vi "MultirunBuilderForNamedLocations3.vi"() -> ()   [LabVIEW 2015]
uses:
  MultirunBuilderSubVIs/RowTemplate.ctl
  Anemometry Sub Vis/Gen Trav/Spacing.ctl
  Anemometry Sub Vis/Controls/Multi_run_mode.ctl
  MultirunBuilderSubVIs/ReformattedTaskArray.ctl
  Anemometry Sub Vis/Controls/Tunnel_Coordinates.ctl
  MultirunBuilderSubVIs/Set Speed Only.vi
  MultirunBuilderSubVIs/Wait (minutes).vi
  MultirunBuilderSubVIs/Single Measurement.vi
  MultirunBuilderSubVIs/Auto Calibrate.vi
  MultirunBuilderSubVIs/MoveTT.vi
  Anemometry Sub Vis/Globals/Meas_global.vi
  Anemometry Sub Vis/File/Setup_Filetype.ctl
panel:
  in  "Generate Cmd File":bool
  in  "Tab Control":enum32{"Globals", "Task Array", "Dev"}(tab)
  in  "TaskArray":T1 {"Carrier_2 Q (l/min)" format="%#.2f"; "Row Duration (mins)" format="%#.1f min"; "Row No" min=0 format="row %.0f"; "Trace Gas Concentration (%)" min=0.0 format="%#_4f"; "Carrier_1 Q (l/min)" format="%#.2f"; "Tunnel Speed" format="%#.2f m/s"; "Start X" format="%#.2f"; "Start Y" format="%#.2f"; "Start Z" format="%#.2f"; "End X" format="%#.2f"; "End Y" format="%#.2f"; "End Z" format="%#.2f"; "No. of pts." format="%.0f pts"; "Averaging time (min)" min=0.0 format="%#.2f min"}
  out "Startup Index":bool
  in  "Re-initialize":bool
  in  "Stop Button":bool
  in  "RowTemplate":T3 {"Carrier_2 Q (l/min)" format="%#.2f"; "Row Duration (mins)" format="%#.1f"; "Row No" min=0; "Trace Gas Concentration (%)" min=0.0 format="%#_4f"; "Carrier_1 Q (l/min)" format="%#.2f"; "Tunnel Speed" format="%#.2f"; "Start X" format="%#.2f"; "Start Y" format="%#.2f"; "Start Z" format="%#.2f"; "End X" format="%#.2f"; "End Y" format="%#.2f"; "End Z" format="%#.2f"; "Averaging time (min)" min=0.0 format="%#.2f"}
  # "X           Y            Z"
  # "Start"
  # "End"
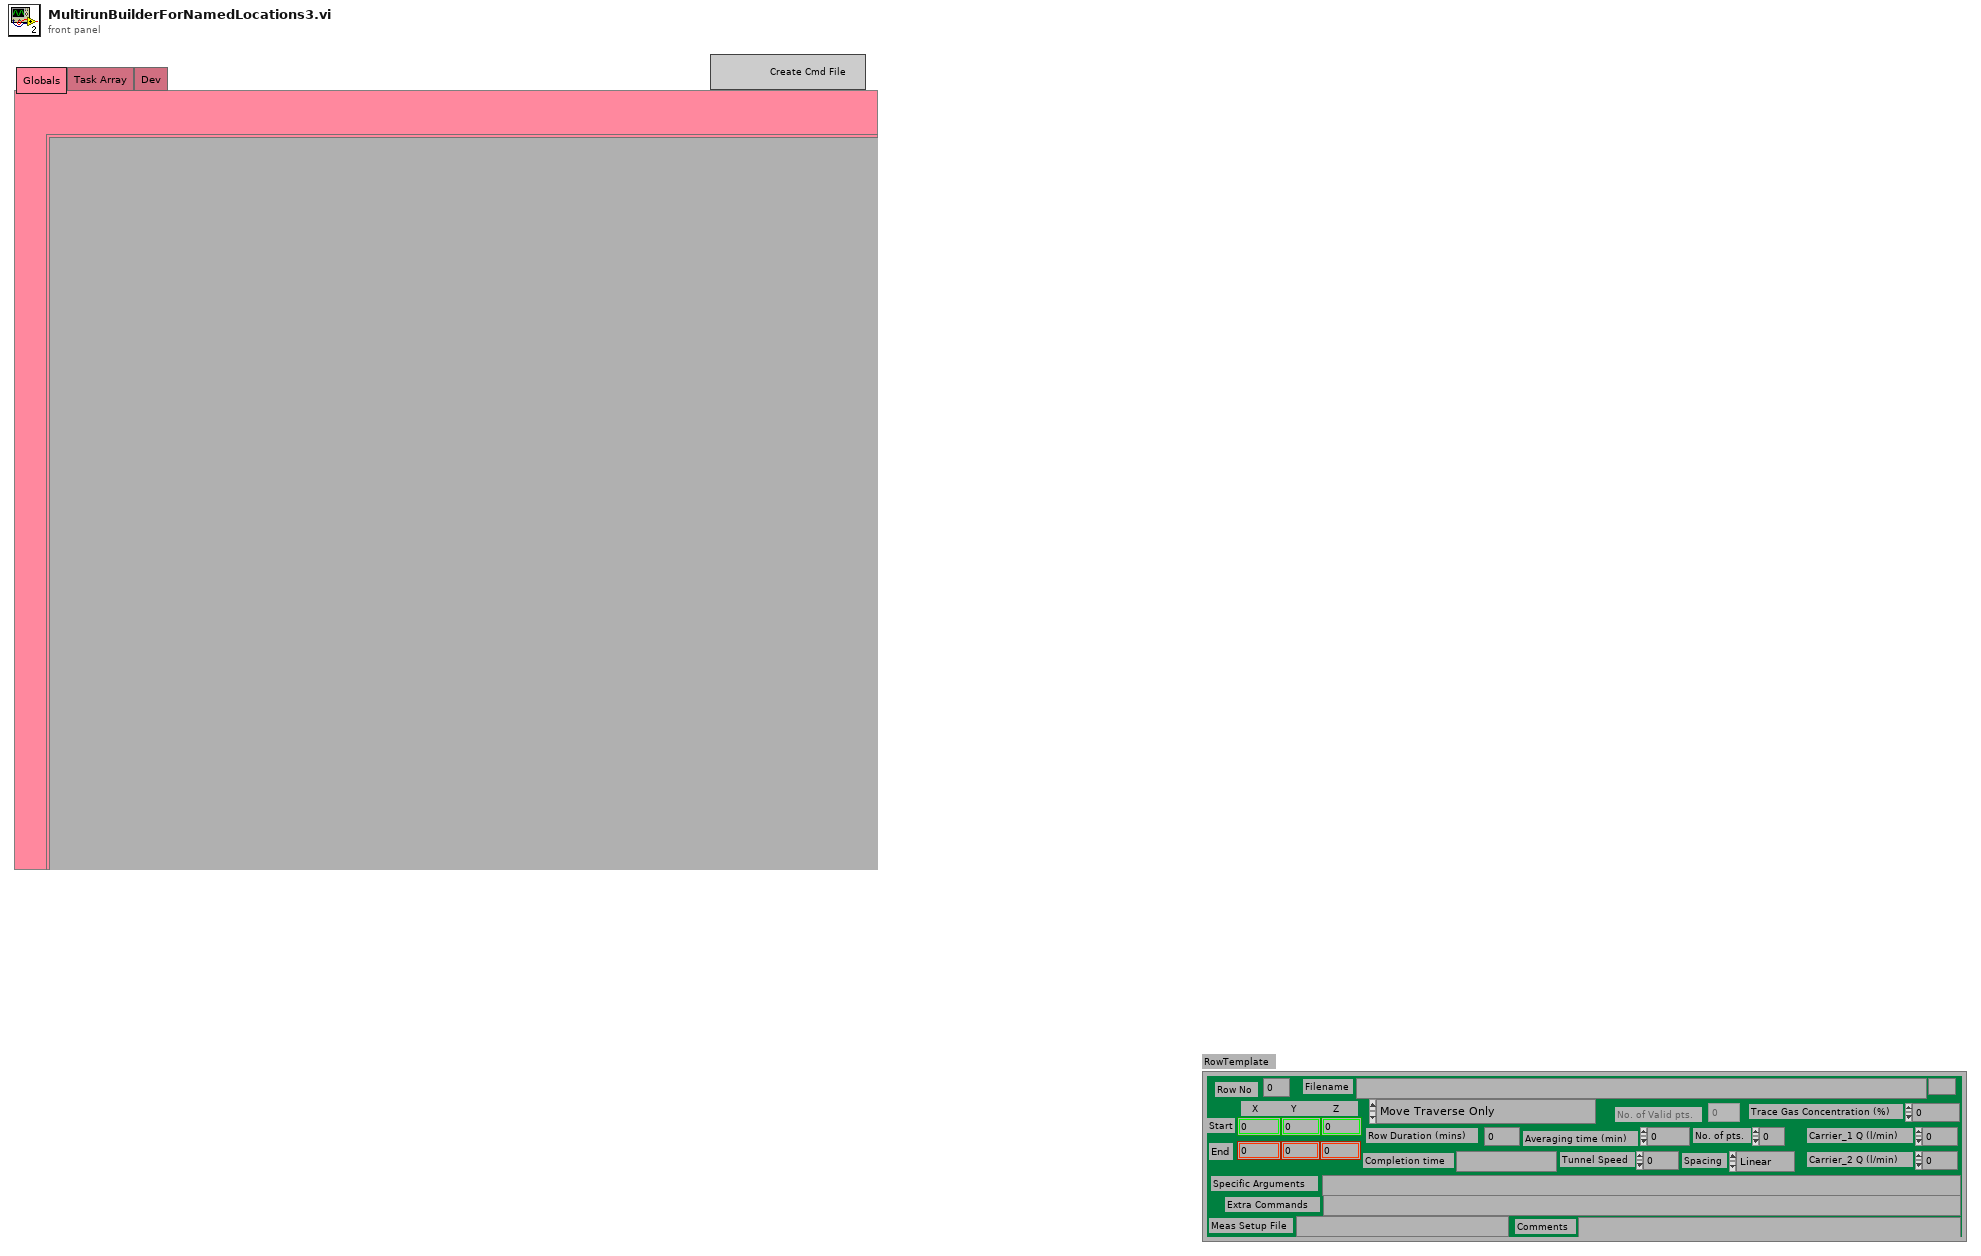
[diagram p1: front panel]
types:
  T1 = typedef "ReformattedTaskArray.ctl" = cluster{"Start X":sgl, "Start Y":sgl, "Start Z":sgl, "End X":sgl, "End Y":sgl, "End Z":sgl, "No. of pts.":i32, "Spacing":T2, "Filename":path, "Tunnel Speed":dbl, "Averaging time (min)":dbl, "Extra Commands":string, "Carrier_1 Q (l/min)":dbl, "Carrier_2 Q (l/min)":dbl, "Trace Gas Concentration (%)":dbl, "Specific Arguments":string, "Comments":string, "Row No":i32, "Row Type Selector":enum16{"Move Traverse Only", "Set Tunnel Speed Only", "Set Source Only", "Set Measurement Conditions", "Single Measurement", "Vertical Profile", "Lateral Profile", "Longitudinal Profile", "Explore Volume", "Multi-Axis Profile", "Auto Calibrate", "Meas Fast FID Bkgnd", "Check Beam Power", "Scanning Valve Measurement", "Run VI Named:", "Set ADAM Ch", "Wait (minutes)", "Send Message", "Synchronize With:", "Fall Back to this Row", "Turn Off Row Repeating", "Blank Row", "Traverse 3D Volume"}, "Completion time":string, "Row Duration (mins)":dbl, "No. of Valid pts.":i32, "Meas Setup File":string}[]
  T2 = typedef "Spacing.ctl" = enum16{"Linear", "Log", "Gauss", "Specified", "N/A"}
  T3 = typedef "RowTemplate.ctl" = cluster{"Start X":sgl, "Start Y":sgl, "Start Z":sgl, "End X":sgl, "End Y":sgl, "End Z":sgl, "No. of pts.":i32, "Spacing":T2, "Filename":path, "Tunnel Speed":dbl, "Averaging time (min)":dbl, "Extra Commands":string, "Carrier_1 Q (l/min)":dbl, "Carrier_2 Q (l/min)":dbl, "Trace Gas Concentration (%)":dbl, "Specific Arguments":string, "Comments":string, "Row No":i32, "Row Type Selector":T4, "Completion time":string, "Row Duration (mins)":dbl, "No. of Valid pts.":i32, "Meas Setup File":string}
  T4 = typedef "Multi_run_mode.ctl" = enum16{"Move Traverse Only", "Set Tunnel Speed Only", "Set Source Only", "Set Measurement Conditions", "Single Measurement", "Vertical Profile", "Lateral Profile", "Longitudinal Profile", "Explore Volume", "Multi-Axis Profile", "Auto Calibrate", "Meas Fast FID Bkgnd", "Check Beam Power", "Scanning Valve Measurement", "Run VI Named:", "Set ADAM Ch", "Wait (minutes)", "Send Message", "Synchronize With:", "Fall Back to this Row", "Turn Off Row Repeating", "Blank Row", "Traverse 3D Volume"}
  T5 = cluster{"Azimuth Array Index":u32, "Vert Prof Array Index":u32, "Lat Prof Array Index":u32, "Azimuth Array Index 2":u32}
  T6 = cluster{"X":dbl, "Y":dbl, "Z":dbl, string, "Use Tunnel Coords?":bool}
  T7 = enum16{"Load Command File", "Save Command File", "Check Multi Run Prog", "Check Multi Run Prog With Live Moves", "Run Multi Run Prog"}
  T8 = typedef "Tunnel_Coordinates.ctl" = enum16{"Work in Tunnel Coordinates", "Work in Model Coordinates"}
  T9 = cluster{"Tunnel Warm Up":bool, "AutoCal":bool, "Zeroes 2":bool, "Turn Table Schedule":bool, "Global Cal Checks":bool, "Local Cal Checks":bool, "Vertical Profile":bool, "Lateral Profile":bool, "Reinitialize Task Array":bool, "Save Command File":bool, "Longitudinal Profile":bool}
  T10 = typedef "CorrectionsCluster.ctl" = cluster{"Use Height Corrections":bool, "TT.Azimuths":dbl[], "Z.HeightCorrs":dbl[][], "Corrections from File":bool, "Height Survey Filepaths":path[]}
  T11 = cluster{"Start X":sgl, "Start Y":sgl, "Start Z":sgl, "End X":sgl, "End Y":sgl, "End Z":sgl, "No. of pts.":i32, "Spacing":T2, "Filename":path, "Tunnel Speed":dbl, "Averaging time (min)":dbl, "Extra Commands":string, "Carrier_1 Q (l/min)":dbl, "Carrier_2 Q (l/min)":dbl, "Trace Gas Concentration (%)":dbl, "Specific Arguments":string, "Comments":string, "Row No":i32, "Row Type Selector":T4, "Completion time":string, "Row Duration (mins)":dbl, "No. of Valid pts.":i32, "Meas Setup File":string}[]
  T12 = typedef "SingleMeas_Repeater.ctl" = cluster{"X":dbl, "Y":dbl, "Z":dbl, "Use Tunnel Coords?":bool, "RepeatEveryXDeg":dbl}
  T13 = typedef "MRBRowTaskSelector.ctl" = enum16{"Move Traverse Only", "Set Tunnel Speed Only", "Set Source Only", "Set Measurement Conditions", "Single Measurement", "Vertical Profile", "Lateral Profile", "Longitudinal Profile", "Explore Volume", "Multi-Axis Profile", "Auto Calibrate", "Meas Fast FID Bkgnd", "Check Beam Power", "Scanning Valve Measurement", "Run VI Named:", "MoveTT", "TravZSurvey", "Set ADAM Ch", "Wait (minutes)", "Send Message", "Synchronize With:", "Fall Back to this Row", "Turn Off Row Repeating", "Blank Row", "Traverse 3D Volume"}
  T14 = cluster{"Row Type Selector":T13, "Index":dbl, "Direction":enum16{"Forward", "Reverse"}}[]
  T15 = cluster{"Tunnel Off":bool, "Local Cal Checks":bool, "Global Cal Checks":bool, "Zeroes":bool, "AutoCal":bool, "Turn Table --> Zero":bool}
  T16 = typedef "Setup_Filetype.ctl" = enum16{"Measurement Setups", "Calibration Setups", "General", "Results File Plotter Setups", "Speed Calib Tweaks"}
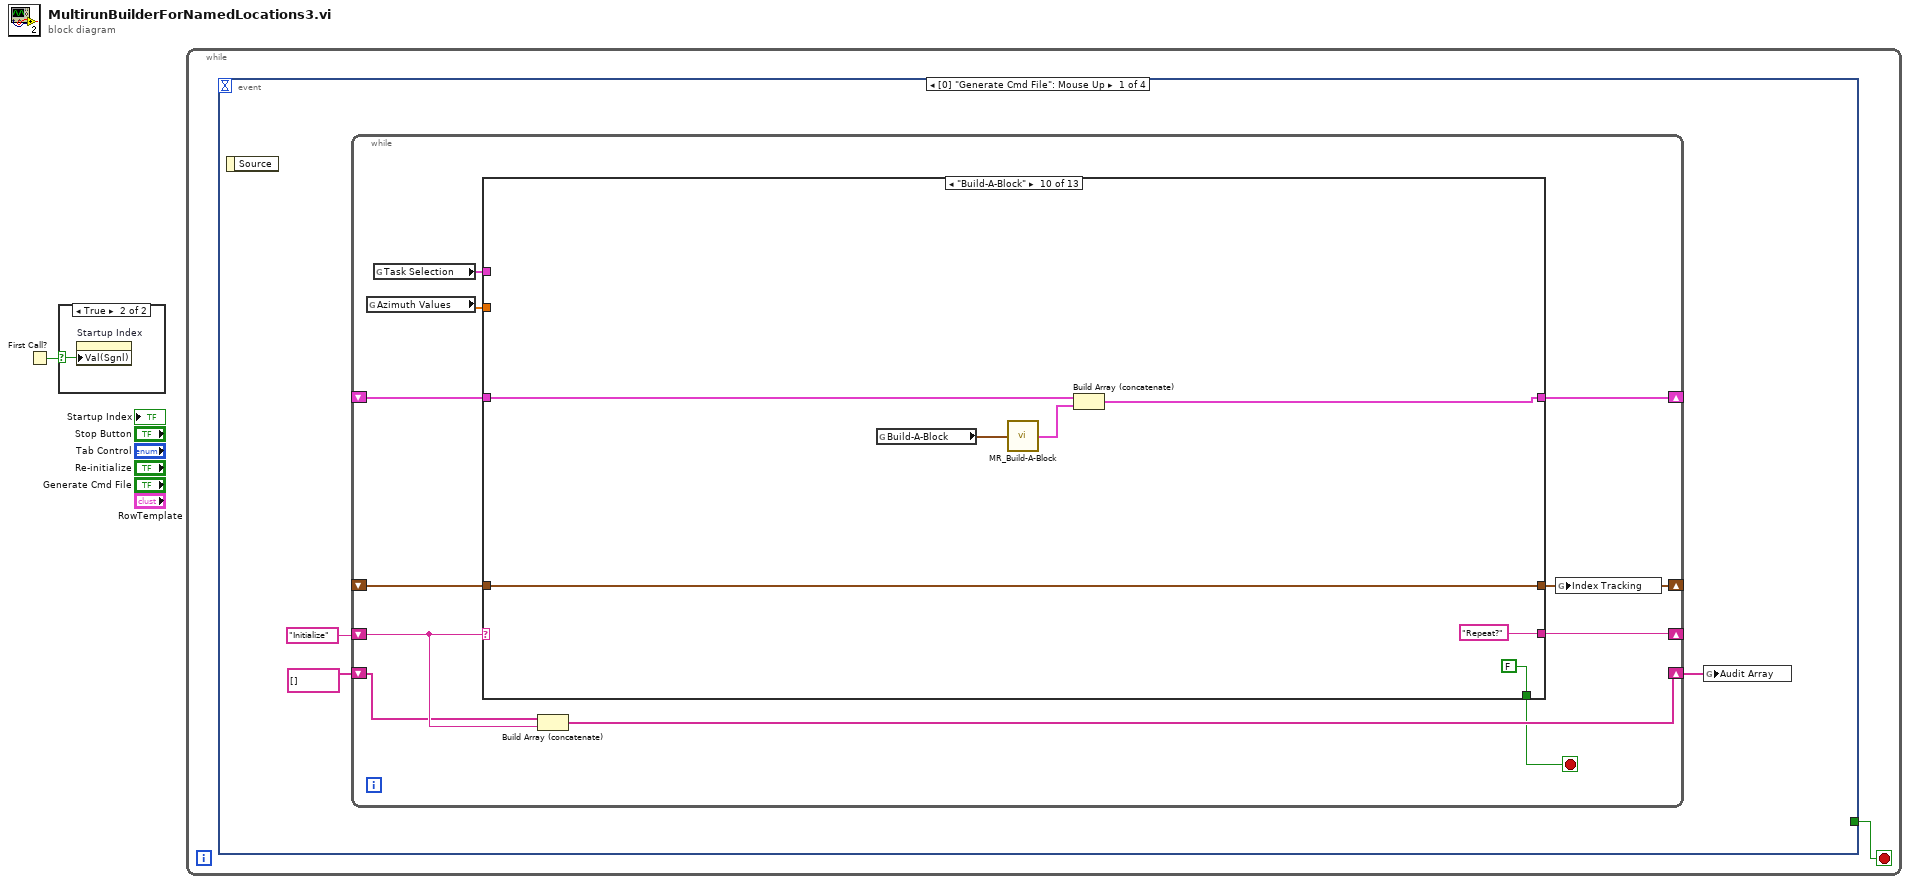
[diagram p0: block diagram]
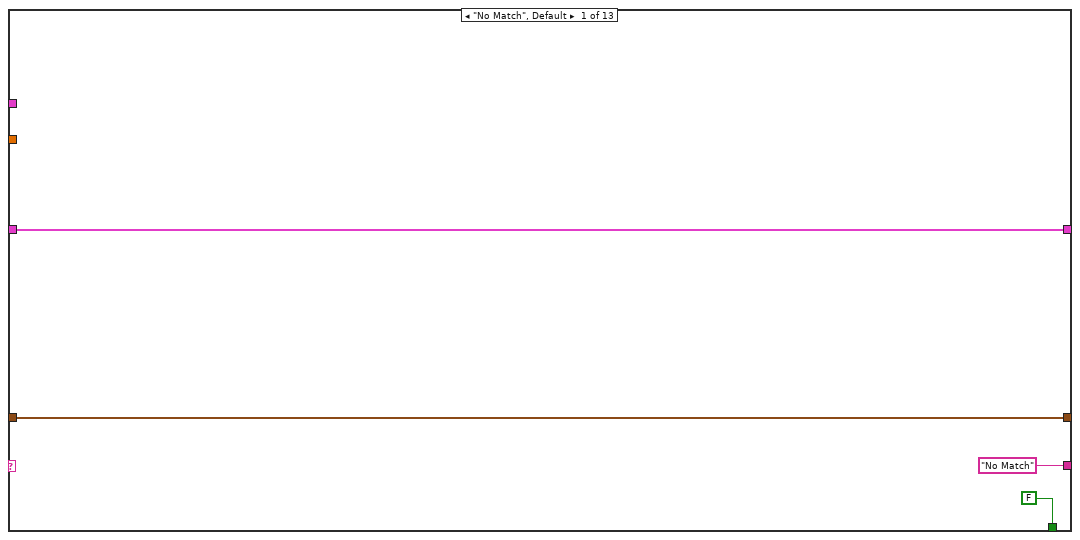
[diagram p2: hidden frame]
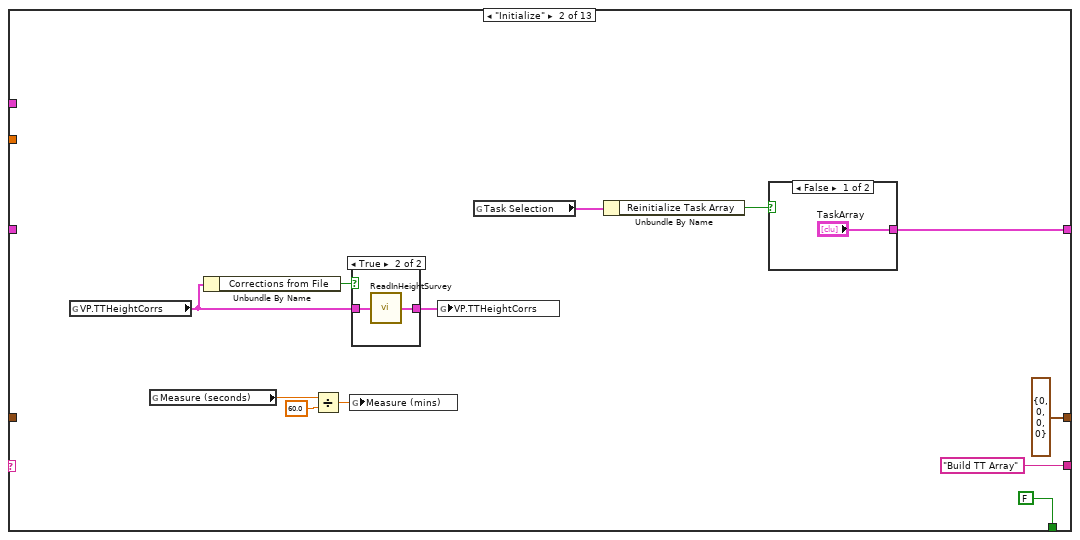
[diagram p3: hidden frame]
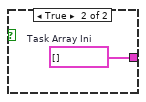
[diagram p5: hidden frame]
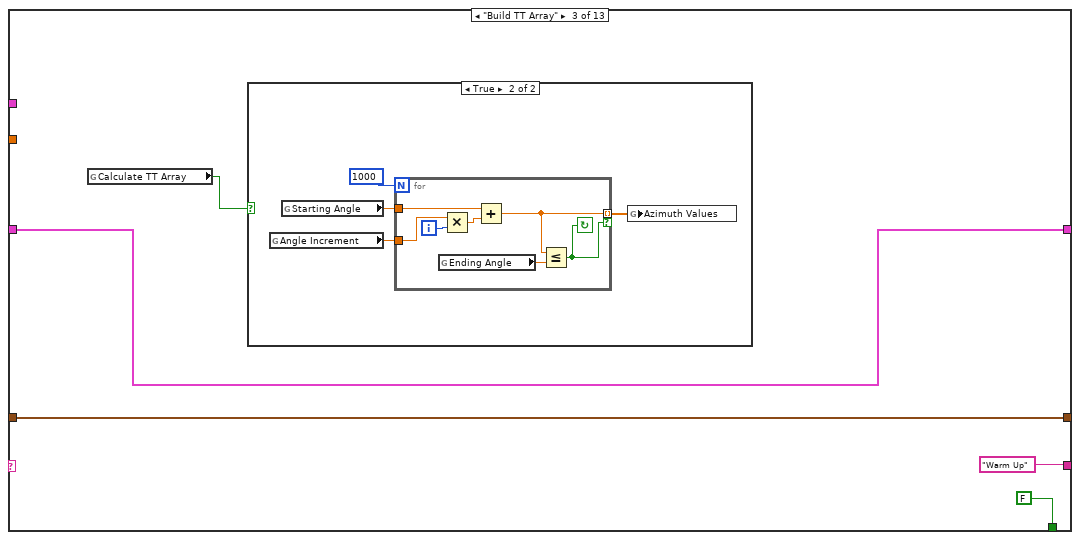
[diagram p6: hidden frame]
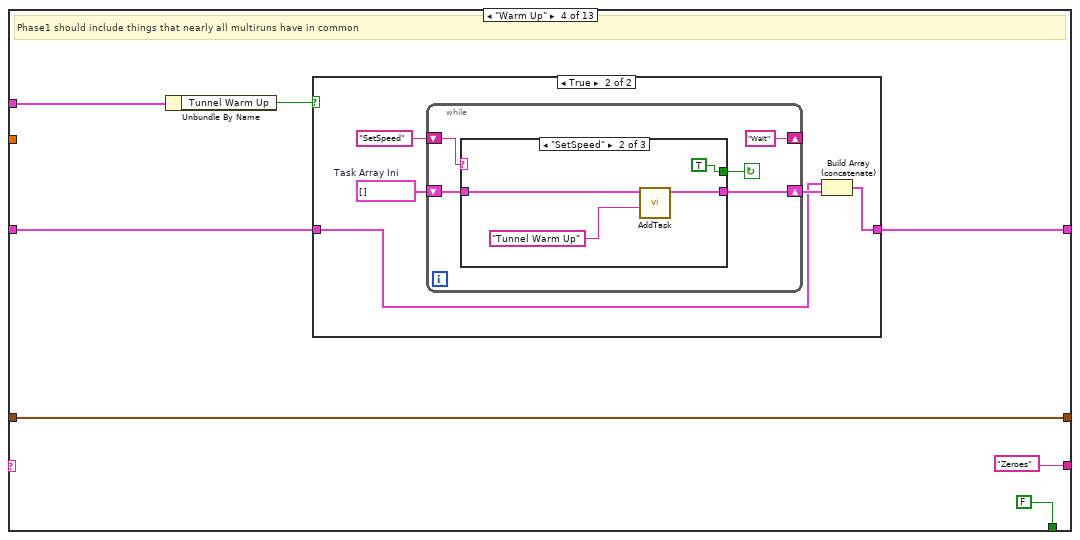
[diagram p8: hidden frame]
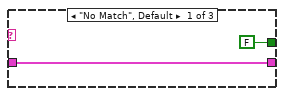
[diagram p10: hidden frame]
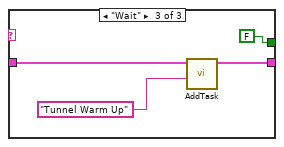
[diagram p11: hidden frame]
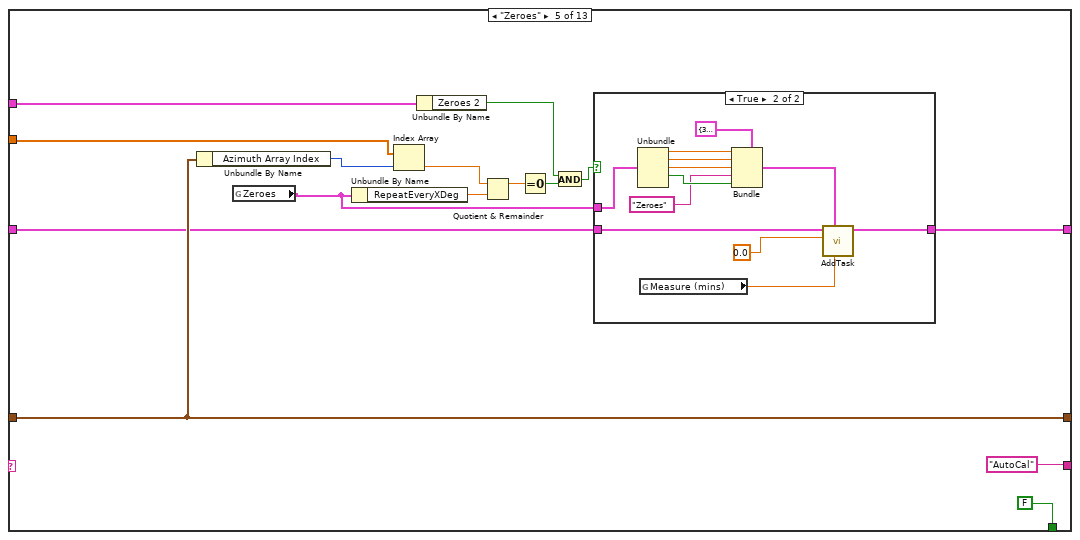
[diagram p12: hidden frame]
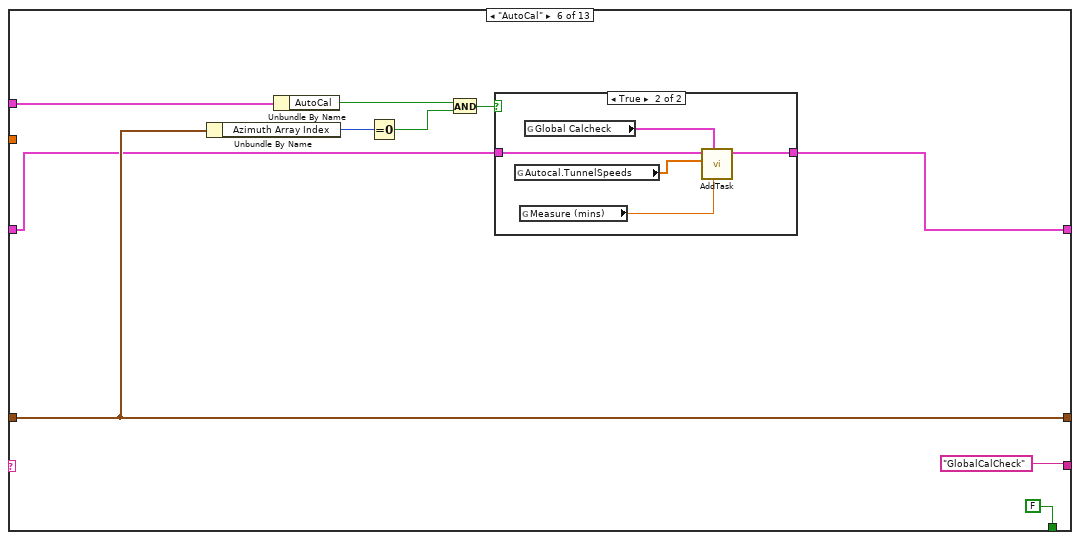
[diagram p14: hidden frame]
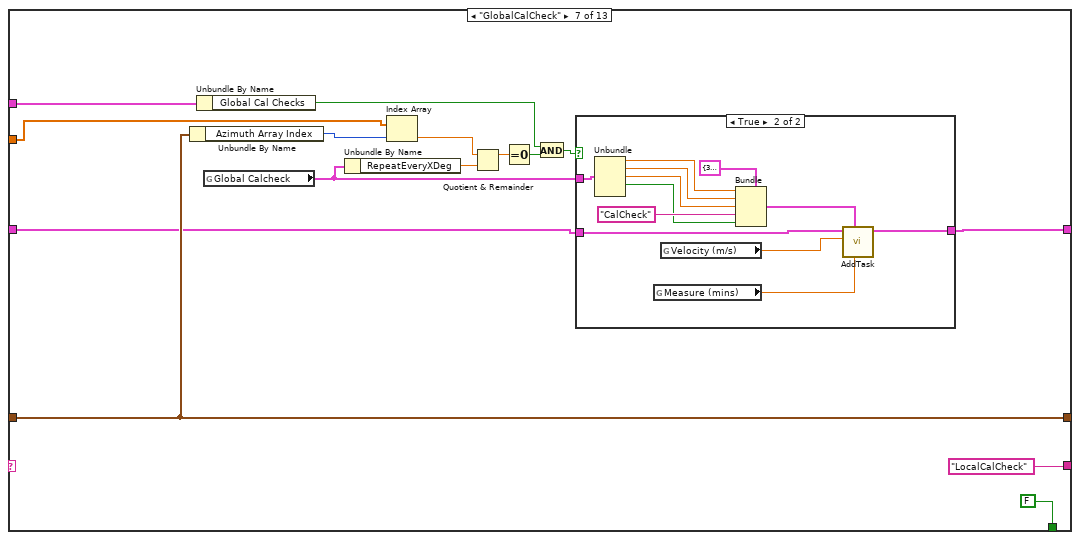
[diagram p16: hidden frame]
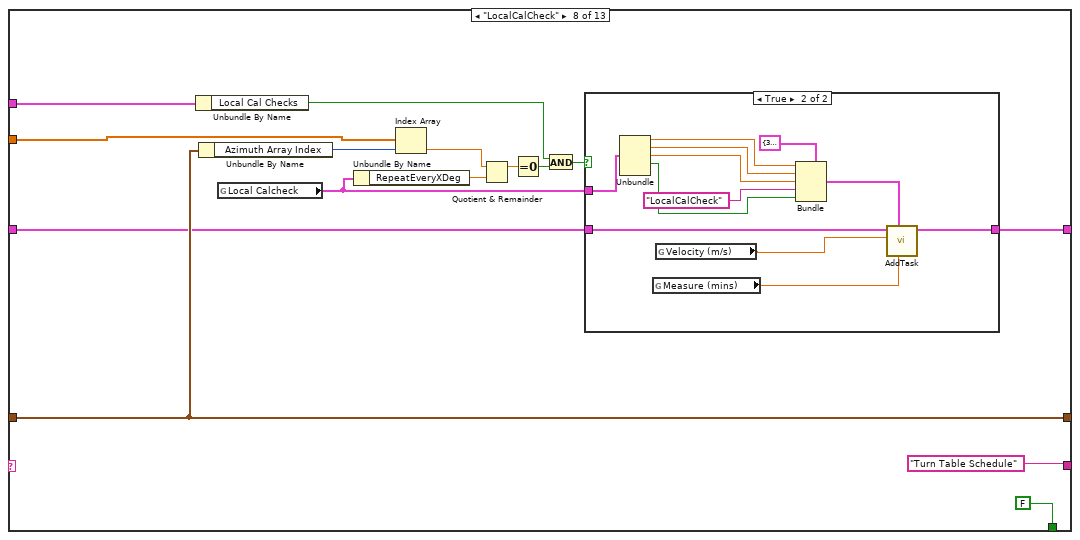
[diagram p18: hidden frame]
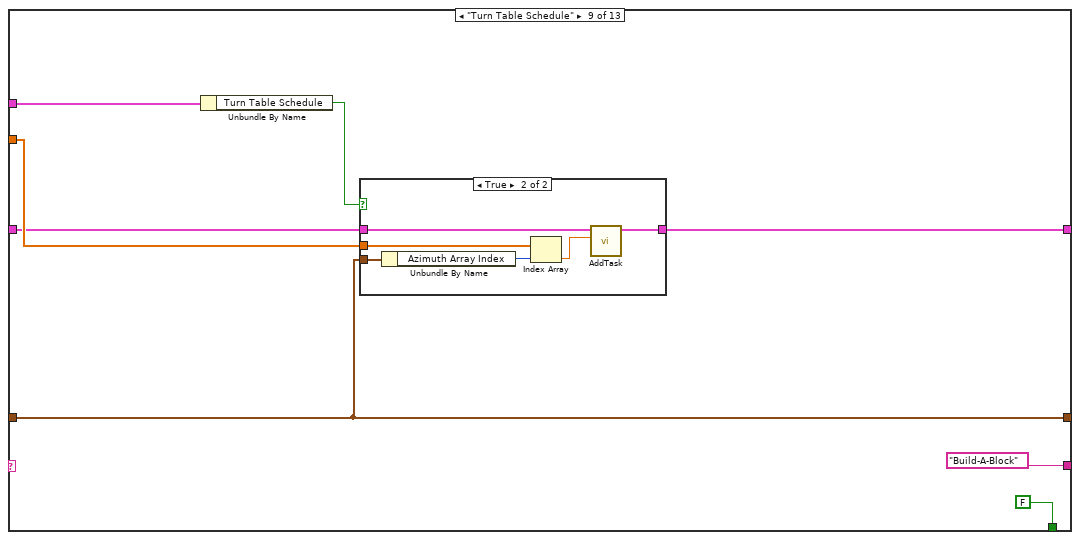
[diagram p20: hidden frame]
diagram:
  n1 = First Call?() -> (First Call?: T/F=w1:bool)
  n2 = case shown="True" w1 {
    selector: w1 -> [_ w2]
    frame False {
    }
    frame True {
      n3 = property on="Startup Index" class="Bool (strict)"("Val(Sgnl)"=w2) -> ()  [unwired: 2 in, 2 out]
    }
  }
  n4 = while {
    stop <- w3 stop-if-true
    n5 = event shown="[0] \"Generate Cmd File\": Mouse Up" {
      selector: _ -> [_ _ _ _]
      dyn-events: _ -> [_ _ _ _]
      timeout: _ -> [_ _ _ _]
      tunnel: [_ _ _ TRUE] -> w3
      event "Generate Cmd File": Mouse Up {
        n6 = event-data() -> ()  [unwired: 1 in, 1 out]
        n7 = while {
          shift-right: [w17] -> _
          shift-left: "Initialize" -> [w15]
          shift-right: [w10] -> _
          shift-left: _ -> [w11]
          shift-right: [w14] -> w6
          shift-left: string[] [] -> [w13]
          shift-right: [w9] -> _
          shift-left: _ -> [w16]
          stop <- w12 stop-if-true
          n8 = global read "MRCMDFBGlobal.vi" "Azimuth Values"() -> (w7:dbl[])
          n9 = global read "MRCMDFBGlobal.vi" "Task Selection"() -> (w8:T9)
          n10 = case shown="\"Build-A-Block\"" w15 {
            tunnel: ["No Match" "Build TT Array" "Warm Up" "Zeroes" "AutoCal" "GlobalCalCheck" "LocalCalCheck" "Turn Table Schedule" "Build-A-Block" "Repeat?" w209 "Save Multirun?" ("t") _] -> w17
            tunnel: [FALSE ("Stop Button") FALSE ("Stop Button") FALSE ("Stop Button") FALSE ("Stop Button") FALSE ("Stop Button") FALSE ("Stop Button") FALSE ("Stop Button") FALSE ("Stop Button") FALSE ("Stop Button") FALSE ("Stop Button") FALSE ("Stop Button") FALSE TRUE] -> w12
            tunnel: w7 -> [_ _ _ _ w95 _ w131 w158 w189 _ w208 _ _]
            tunnel: w16 -> [w19 _ w42 w59 w93 w117 w134 w163 w185 w199 w214 w242 w342]
            tunnel: [w19 T5 {"Azimuth Array Index"=0, "Vert Prof Array Index"=0, "Lat Prof Array Index"=0, "Azimuth Array Index 2"=0} ("Index Tracking") w42 w59 w93 w117 w134 w163 w185 w199 w212 w242 w342] -> w9
            tunnel: w8 -> [_ _ _ w58 w89 w113 w133 w162 w186 _ w205 _ w346]
            tunnel: w11 -> [w18 _ w40 w56 w84 w111 w128 w157 w184 w201 w206 w233 w344]
            tunnel: [w18 w28 w40 w55 w85 w112 w129 w156 w183 w200 w206 w234 w340] -> w10
            frame "No Match", Default {
            }
            frame "Initialize" {
              n11 = global read "MRCMDFBGlobal.vi" "VP.TTHeightCorrs"() -> (w25:T10)
              n12 = global read "MRCMDFBGlobal.vi" "Measure (seconds)"() -> (w22:dbl)
              n13 = Unbundle By Name(w25) -> ("Corrections from File"=w27:bool)
              n14 = Divide(x=w22, y=60.0 ("x")) -> (x/y=w23:dbl)
              n15 = global write "MRCMDFBGlobal.vi" "Measure (mins)"(w23) -> ()
              n16 = case shown="True" w27 {
                tunnel: w25 -> [w34 w36]
                tunnel: [w34 w35] -> w26
                frame False {
                }
                frame True {
                  n17 = call "ReadInHeightSurvey.vi"("VP.TTHeightCorrs In"=w36) -> ("VP.TTHeightCorrs Out"=w35:T10)
                }
              }
              n18 = global write "MRCMDFBGlobal.vi" "VP.TTHeightCorrs"(w26) -> ()
              n19 = global read "MRCMDFBGlobal.vi" "Task Selection"() -> (w30:T9)
              n20 = Unbundle By Name(w30) -> ("Reinitialize Task Array"=w29:bool)
              n21 = case shown="False" w29 {
                tunnel: ["TaskArray" w38] -> w28
                frame False {
                }
                frame True {
                  w38 = T11 []  # Task Array Ini
                }
              }
            }
            frame "Build TT Array" {
              n22 = global read "MRCMDFBGlobal.vi" "Calculate TT Array"() -> (w39:bool)
              n23 = case shown="True" w39 {
                frame False {
                }
                frame True {
                  n24 = global read "MRCMDFBGlobal.vi" "Angle Increment"() -> (w44:dbl)
                  n25 = global read "MRCMDFBGlobal.vi" "Starting Angle"() -> (w45:dbl)
                  n26 = for {
                    N: 1000 -> [_]
                    tunnel: w45 -> [w52]
                    tunnel: w44 -> [w53]
                    tunnel: [w50] -> w46 mode=indexing if=w49
                    i -> [w54]
                    stop <- w49 continue-if-true
                    n27 = global read "MRCMDFBGlobal.vi" "Ending Angle"() -> (w48:dbl)
                    n28 = Multiply(x=w53, y=w54) -> (x*y=w51:dbl)
                    n29 = Add(x=w52, y=w51) -> (x+y=w50:dbl)
                    n30 = Less Or Equal?(x=w50, y=w48) -> (x <= y?=w49:bool)
                  }
                  n31 = global write "MRCMDFBGlobal.vi" "Azimuth Values"(w46) -> ()
                }
              }
            }
            frame "Warm Up" {
              # "Phase1 should include things that nearly all multiruns have in common"
              n32 = Unbundle By Name(w58) -> ("Tunnel Warm Up"=w57:bool)
              n33 = case shown="True" w57 {
                tunnel: w56 -> [w62 w64]
                tunnel: [w62 w63] -> w55
                frame False {
                }
                frame True {
                  w66 = T11 []  # Task Array Ini
                  n34 = while {
                    shift-right: ["Wait"] -> _
                    shift-left: "SetSpeed" -> [w72]
                    shift-right: [w68] -> w65
                    shift-left: w66 -> [w69]
                    stop <- w70 continue-if-true
                    n35 = case shown="\"SetSpeed\"" w72 {
                      tunnel: [FALSE TRUE FALSE] -> w70
                      tunnel: w69 -> [w73 w76 w80]
                      tunnel: [w73 w75 w79] -> w68
                      frame "No Match", Default {
                      }
                      frame "SetSpeed" {
                        n36 = call-poly "AddTask.vi"("Comments"="Tunnel Warm Up", "Input Task Array"=w76) -> ("Output Task Array"=w75:T3[])  [unwired: 9 in]
                      }
                      frame "Wait" {
                        n37 = call-poly "AddTask.vi"("Comments"="Tunnel Warm Up", "Input Task Array"=w80) -> ("Output Task Array"=w79:T3[])  [unwired: 9 in]
                      }
                    }
                  }
                  n38 = Build Array (concatenate)(w64, w65) -> (w63:T3[])
                }
              }
            }
            frame "Zeroes" {
              n39 = Unbundle By Name(w93) -> ("Azimuth Array Index"=w94:u32)
              n40 = global read "MRCMDFBGlobal.vi" "Zeroes"() -> (w83:T12)
              n41 = Unbundle By Name(w83) -> ("RepeatEveryXDeg"=w91:dbl)
              n42 = Index Array(array=w95, index=w94) -> (element=w92:dbl)
              n43 = Unbundle By Name(w89) -> ("Zeroes 2"=w88:bool)
              n44 = Quotient & Remainder(x=w92, y=w91) -> (x-y*floor(x/y)=w90:dbl)  [unwired: 1 out]
              n45 = Equal To 0?(x=w90) -> (x = 0?=w87:bool)
              n46 = And(x=w88, y=w87) -> (x .and. y?=w86:bool)
              n47 = case shown="True" w86 {
                tunnel: w83 -> [_ w107]
                tunnel: [w98 w109] -> w85
                tunnel: w84 -> [w98 w108]
                frame False {
                }
                frame True {
                  n48 = Unbundle(w107) -> ("X"=w105:dbl, "Y"=w104:dbl, "Z"=w103:dbl, "Use Tunnel Coords?"=w101:bool)  [unwired: 1 out]
                  n49 = global read "MRCMDFBGlobal.vi" "Measure (mins)"() -> (w99:dbl)
                  n50 = Bundle(cluster=T6 {"X"=36.0, "Y"=54.0, "Z"=300.0, "", "Use Tunnel Coords?"=TRUE} ("Coordinate Location"), "X"=w105, "Y"=w104, "Z"=w103, "Zeroes" ("Comments"), "Use Tunnel Coords?"=w101) -> (w102:T6)
                  n51 = call-poly "AddTask.vi"("Averaging time (min)"=w99, "Coordinate Description"=w102, "Tunnel Speed"=0.0, "Input Task Array"=w108) -> ("Output Task Array"=w109:T3[])  [unwired: 7 in]
                }
              }
            }
            frame "AutoCal" {
              n52 = Unbundle By Name(w117) -> ("Azimuth Array Index"=w116:u32)
              n53 = Unbundle By Name(w113) -> ("AutoCal"=w115:bool)
              n54 = Equal To 0?(x=w116) -> (x = 0?=w118:bool)
              n55 = And(x=w115, y=w118) -> (x .and. y?=w114:bool)
              n56 = case shown="True" w114 {
                tunnel: [w121 w126] -> w112
                tunnel: w111 -> [w121 w125]
                frame False {
                }
                frame True {
                  n57 = global read "MRCMDFBGlobal.vi" "Autocal.TunnelSpeeds"() -> (w124:dbl[])
                  n58 = global read "MRCMDFBGlobal.vi" "Measure (mins)"() -> (w123:dbl)
                  n59 = global read "MRCMDFBGlobal.vi" "Global Calcheck"() -> (w122:T12)
                  n60 = call-poly "AddTask.vi"("Averaging time (min)"=w123, "Global Calcheck"=w122, "Autocal.TunnelSpeeds"=w124, "Input Task Array"=w125) -> ("Output Task Array"=w126:T3[])  [unwired: 7 in]
                }
              }
            }
            frame "GlobalCalCheck" {
              n61 = Unbundle By Name(w134) -> ("Azimuth Array Index"=w139:u32)
              n62 = Unbundle By Name(w133) -> ("Global Cal Checks"=w132:bool)
              n63 = global read "MRCMDFBGlobal.vi" "Global Calcheck"() -> (w127:T12)
              n64 = Unbundle By Name(w127) -> ("RepeatEveryXDeg"=w137:dbl)
              n65 = Index Array(array=w131, index=w139) -> (element=w138:dbl)
              n66 = Quotient & Remainder(x=w138, y=w137) -> (x-y*floor(x/y)=w136:dbl)  [unwired: 1 out]
              n67 = Equal To 0?(x=w136) -> (x = 0?=w135:bool)
              n68 = And(x=w132, y=w135) -> (x .and. y?=w130:bool)
              n69 = case shown="True" w130 {
                tunnel: w127 -> [_ w152]
                tunnel: [w142 w154] -> w129
                tunnel: w128 -> [w142 w153]
                frame False {
                }
                frame True {
                  n70 = Unbundle(w152) -> ("X"=w149:dbl, "Y"=w148:dbl, "Z"=w147:dbl, "Use Tunnel Coords?"=w146:bool)  [unwired: 1 out]
                  n71 = global read "MRCMDFBGlobal.vi" "Measure (mins)"() -> (w143:dbl)
                  n72 = global read "MRCMDFBGlobal.vi" "Velocity (m/s)"() -> (w144:dbl)
                  n73 = Bundle(cluster=T6 {"X"=36.0, "Y"=54.0, "Z"=300.0, "", "Use Tunnel Coords?"=TRUE} ("Coordinate Location"), "X"=w149, "Y"=w148, "Z"=w147, "CalCheck" ("Comments"), "Use Tunnel Coords?"=w146) -> (w145:T6)
                  n74 = call-poly "AddTask.vi"("Averaging time (min)"=w143, "Coordinate Description"=w145, "Tunnel Speed"=w144, "Input Task Array"=w153) -> ("Output Task Array"=w154:T3[])  [unwired: 7 in]
                }
              }
            }
            frame "LocalCalCheck" {
              n75 = Unbundle By Name(w162) -> ("Local Cal Checks"=w161:bool)
              n76 = Unbundle By Name(w163) -> ("Azimuth Array Index"=w167:u32)
              n77 = global read "MRCMDFBGlobal.vi" "Local Calcheck"() -> (w155:T12)
              n78 = Unbundle By Name(w155) -> ("RepeatEveryXDeg"=w165:dbl)
              n79 = Index Array(array=w158, index=w167) -> (element=w166:dbl)
              n80 = Quotient & Remainder(x=w166, y=w165) -> (x-y*floor(x/y)=w164:dbl)  [unwired: 1 out]
              n81 = Equal To 0?(x=w164) -> (x = 0?=w160:bool)
              n82 = And(x=w161, y=w160) -> (x .and. y?=w159:bool)
              n83 = case shown="True" w159 {
                tunnel: w155 -> [_ w180]
                tunnel: w157 -> [w170 w182]
                tunnel: [w170 w181] -> w156
                frame False {
                }
                frame True {
                  n84 = Unbundle(w180) -> ("X"=w173:dbl, "Y"=w174:dbl, "Z"=w175:dbl, "Use Tunnel Coords?"=w176:bool)  [unwired: 1 out]
                  n85 = global read "MRCMDFBGlobal.vi" "Measure (mins)"() -> (w171:dbl)
                  n86 = global read "MRCMDFBGlobal.vi" "Velocity (m/s)"() -> (w172:dbl)
                  n87 = Bundle(cluster=T6 {"X"=36.0, "Y"=54.0, "Z"=300.0, "", "Use Tunnel Coords?"=TRUE} ("Coordinate Location"), "X"=w173, "Y"=w174, "Z"=w175, "LocalCalCheck" ("Comments"), "Use Tunnel Coords?"=w176) -> (w177:T6)
                  n88 = call-poly "AddTask.vi"("Averaging time (min)"=w171, "Coordinate Description"=w177, "Tunnel Speed"=w172, "Input Task Array"=w182) -> ("Output Task Array"=w181:T3[])  [unwired: 7 in]
                }
              }
            }
            frame "Turn Table Schedule" {
              n89 = Unbundle By Name(w186) -> ("Turn Table Schedule"=w187:bool)
              n90 = case shown="True" w187 {
                tunnel: w189 -> [_ w197]
                tunnel: w185 -> [_ w196]
                tunnel: w184 -> [w191 w195]
                tunnel: [w191 w194] -> w183
                frame False {
                }
                frame True {
                  n91 = Unbundle By Name(w196) -> ("Azimuth Array Index"=w193:u32)
                  n92 = Index Array(array=w197, index=w193) -> (element=w192:dbl)
                  n93 = call-poly "AddTask.vi"("TT:Azimuth"=w192, "Input Task Array"=w195) -> ("Output Task Array"=w194:T3[])  [unwired: 9 in]
                }
              }
            }
            frame "Build-A-Block" {
              n94 = global read "MRCMDFBGlobal.vi" "Build-A-Block"() -> (w198:T14)
              n95 = call "MR_Build-A-Block.vi"("Build-A-Block"=w198) -> ("TaskArray"=w202:T11)
              n96 = Build Array (concatenate)(w201, w202) -> (w200:T3[])
            }
            frame "Repeat?" {
              # "Only reason to repeat is if TT Scheduling"
              n97 = Unbundle By Name(w205) -> ("Turn Table Schedule"=w207:bool)
              n98 = case shown="True" w207 {
                tunnel: w214 -> [w216 w223]
                tunnel: [TRUE w222] -> w213
                tunnel: [w216 w221] -> w212
                tunnel: w208 -> [_ w220]
                frame False {
                }
                frame True {
                  n99 = Array Size(array=w220) -> (size(s)=w219:i32)
                  n100 = Decrement(x=w219) -> (x-1=w218:i32)
                  n101 = in-place {
                    in-place-border: w218 -> [w225]
                    in-place-border: [w226] -> w222
                    n102 = in-place-cluster #1(w223) -> ("Azimuth Array Index"=w224:u32)
                    n103 = Equal?(x=w225, y=w224) -> (x = y?=w226:bool)
                    n104 = case shown="True" w226 {
                      tunnel: [w228 0] -> w227
                      tunnel: w224 -> [w229 _]
                      frame False {
                        n105 = Increment(x=w229) -> (x+1=w228:u32)
                      }
                      frame True {
                      }
                    }
                    n106 = in-place-cluster #1("Azimuth Array Index"=w227) -> (w221:T5)
                  }
                }
              }
              n107 = Select(t="End", s=w213, f="Zeroes" ("t")) -> (s? t:f=w209:string)
            }
            frame "End" {
              n108 = global read "MRCMDFBGlobal.vi" "Multirun Closure Tasks"() -> (w231:T15)
              n109 = Unbundle By Name(w231) -> ("Turn Table --> Zero"=w240:bool, "Zeroes"=w239:bool, "AutoCal"=w238:bool, "Global Cal Checks"=w237:bool, "Local Cal Checks"=w236:bool, "Tunnel Off"=w235:bool)
              n110 = while {
                shift-right: [w253] -> _
                shift-left: "Turn Table" -> [w254]
                tunnel: w240 -> [w252]
                tunnel: w239 -> [w249]
                tunnel: w238 -> [w248]
                tunnel: w237 -> [w247]
                tunnel: w236 -> [w246]
                tunnel: w235 -> [w245]
                shift-right: [w250] -> w234
                shift-left: w233 -> [w251]
                stop <- w244 continue-if-true
                n111 = case shown="\"GlobalCalCheck\"" w254 {
                  tunnel: [_ "Zeroes" "AutoCal" "GlobalCalCheck" "LocalCalCheck" "Tunnel Off" _] -> w253
                  tunnel: w252 -> [_ w261 _ _ _ _ _]
                  tunnel: w251 -> [w256 w260 w270 w288 w299 w317 w334]
                  tunnel: [w256 w259 w269 w287 w298 w316 w333] -> w250
                  tunnel: w249 -> [_ _ w266 _ _ _ _]
                  tunnel: w248 -> [_ _ _ w284 _ _ _]
                  tunnel: w247 -> [_ _ _ _ w296 _ _]
                  tunnel: w246 -> [_ _ _ _ _ w314 _]
                  tunnel: w245 -> [_ _ _ _ _ _ w332]
                  tunnel: [FALSE TRUE TRUE TRUE TRUE TRUE TRUE] -> w244
                  frame "No Match", Default {
                  }
                  frame "Turn Table" {
                    n112 = case shown="True" w261 {
                      tunnel: w260 -> [w262 w264]
                      tunnel: [w262 w263] -> w259
                      frame False {
                      }
                      frame True {
                        n113 = call-poly "AddTask.vi"("TT:Azimuth"=0.0, "Input Task Array"=w264) -> ("Output Task Array"=w263:T3[])  [unwired: 9 in]
                      }
                    }
                  }
                  frame "Zeroes" {
                    n114 = case shown="True" w266 {
                      tunnel: w270 -> [w271 w282]
                      tunnel: [w271 w281] -> w269
                      frame False {
                      }
                      frame True {
                        n115 = global read "MRCMDFBGlobal.vi" "Zeroes"() -> (w272:T12)
                        n116 = global read "MRCMDFBGlobal.vi" "Measure (mins)"() -> (w273:dbl)
                        n117 = Unbundle(w272) -> ("X"=w278:dbl, "Y"=w277:dbl, "Z"=w276:dbl, "Use Tunnel Coords?"=w275:bool)  [unwired: 1 out]
                        n118 = Bundle(cluster=T6 {"X"=36.0, "Y"=54.0, "Z"=300.0, "", "Use Tunnel Coords?"=TRUE} ("Coordinate Location"), "X"=w278, "Y"=w277, "Z"=w276, "Zeroes" ("Comments"), "Use Tunnel Coords?"=w275) -> (w274:T6)
                        n119 = call-poly "AddTask.vi"("Averaging time (min)"=w273, "Coordinate Description"=w274, "Tunnel Speed"=0.0, "Input Task Array"=w282) -> ("Output Task Array"=w281:T3[])  [unwired: 7 in]
                      }
                    }
                  }
                  frame "AutoCal" {
                    n120 = case shown="True" w284 {
                      tunnel: w288 -> [w289 w294]
                      tunnel: [w289 w293] -> w287
                      frame False {
                      }
                      frame True {
                        n121 = global read "MRCMDFBGlobal.vi" "Autocal.TunnelSpeeds"() -> (w292:dbl[])
                        n122 = global read "MRCMDFBGlobal.vi" "Global Calcheck"() -> (w290:T12)
                        n123 = global read "MRCMDFBGlobal.vi" "Measure (mins)"() -> (w291:dbl)
                        n124 = call-poly "AddTask.vi"("Averaging time (min)"=w291, "Global Calcheck"=w290, "Autocal.TunnelSpeeds"=w292, "Input Task Array"=w294) -> ("Output Task Array"=w293:T3[])  [unwired: 7 in]
                      }
                    }
                  }
                  frame "GlobalCalCheck" {
                    n125 = case shown="True" w296 {
                      tunnel: w299 -> [w300 w312]
                      tunnel: [w300 w311] -> w298
                      frame False {
                      }
                      frame True {
                        n126 = global read "MRCMDFBGlobal.vi" "Global Calcheck"() -> (w303:T12)
                        n127 = global read "MRCMDFBGlobal.vi" "Measure (mins)"() -> (w301:dbl)
                        n128 = global read "MRCMDFBGlobal.vi" "Velocity (m/s)"() -> (w302:dbl)
                        n129 = Unbundle(w303) -> ("X"=w307:dbl, "Y"=w306:dbl, "Z"=w305:dbl, "Use Tunnel Coords?"=w304:bool)  [unwired: 1 out]
                        n130 = Bundle(cluster=T6 {"X"=36.0, "Y"=54.0, "Z"=300.0, "", "Use Tunnel Coords?"=TRUE} ("Coordinate Location"), "X"=w307, "Y"=w306, "Z"=w305, "CalCheck" ("Comments"), "Use Tunnel Coords?"=w304) -> (w308:T6)
                        n131 = call-poly "AddTask.vi"("Averaging time (min)"=w301, "Coordinate Description"=w308, "Tunnel Speed"=w302, "Input Task Array"=w312) -> ("Output Task Array"=w311:T3[])  [unwired: 7 in]
                      }
                    }
                  }
                  frame "LocalCalCheck" {
                    n132 = case shown="True" w314 {
                      tunnel: w317 -> [w318 w330]
                      tunnel: [w318 w329] -> w316
                      frame False {
                      }
                      frame True {
                        n133 = global read "MRCMDFBGlobal.vi" "Local Calcheck"() -> (w321:T12)
                        n134 = global read "MRCMDFBGlobal.vi" "Measure (mins)"() -> (w319:dbl)
                        n135 = global read "MRCMDFBGlobal.vi" "Velocity (m/s)"() -> (w320:dbl)
                        n136 = Unbundle(w321) -> ("X"=w327:dbl, "Y"=w326:dbl, "Z"=w325:dbl, "Use Tunnel Coords?"=w322:bool)  [unwired: 1 out]
                        n137 = Bundle(cluster=T6 {"X"=36.0, "Y"=54.0, "Z"=300.0, "", "Use Tunnel Coords?"=TRUE} ("Coordinate Location"), "X"=w327, "Y"=w326, "Z"=w325, "LocalCalCheck" ("Comments"), "Use Tunnel Coords?"=w322) -> (w323:T6)
                        n138 = call-poly "AddTask.vi"("Averaging time (min)"=w319, "Coordinate Description"=w323, "Tunnel Speed"=w320, "Input Task Array"=w330) -> ("Output Task Array"=w329:T3[])  [unwired: 7 in]
                      }
                    }
                  }
                  frame "Tunnel Off" {
                    n139 = case shown="True" w332 {
                      tunnel: w334 -> [w335 w337]
                      tunnel: [w335 w336] -> w333
                      frame False {
                      }
                      frame True {
                        n140 = call-poly "AddTask.vi"("Comments"="Tunnel Off", "Tunnel Speed"=0.0, "Input Task Array"=w337) -> ("Output Task Array"=w336:T3[])  [unwired: 8 in]
                      }
                    }
                  }
                }
              }
            }
            frame "Save Multirun?" {
              n141 = Unbundle By Name(w346) -> ("Save Command File"=w345:bool)
              n142 = global read "MRCMDFBGlobal.vi" "Command File Path / Name"() -> (w341:path)
              n143 = case shown="True" w345 {
                tunnel: w341 -> [_ w352]
                tunnel: w344 -> [w347 w349]
                tunnel: [w347 w349] -> w340
                frame False {
                }
                frame True {
                  n144 = global read "MRCMDFBGlobal.vi" "Work in TUNNEL Coordinates"() -> (w348:bool)
                  n145 = case shown="False" w348 {
                    tunnel: [Tunnel_Coordinates."Work in Model Coordinates" ("Work in Tunnel Coordinates?") Tunnel_Coordinates."Work in Tunnel Coordinates" ("Work in Tunnel Coordinates?")] -> w350
                    frame False {
                    }
                    frame True {
                    }
                  }
                  n146 = call "Multi_Run_Prog.vi"("Command filename"=w352, "Mode"=T7."Save Command File", "Table"=w349, "Work in Tunnel Coordinates?"=w350) -> ()  [unwired: 15 in, 1 out]
                }
              }
              n147 = local write "TaskArray"(w340) -> ()
            }
          }
          n148 = Build Array (concatenate)(w13, w15) -> (w14:string[])
          n149 = global write "MRCMDFBGlobal.vi" "Index Tracking"(w9) -> ()
        }
        n150 = global write "MRCMDFBGlobal.vi" "Audit Array"(w6) -> ()
      }
      event "Re-initialize": Mouse Up; "Startup Index": Value Change {
        n151 = event-data() -> ()  [unwired: 1 in, 4 out]
        n152 = while {
          shift-right: [w357] -> _
          shift-left: "Load Subpanel" -> [w358]
          stop <- w356 stop-if-true
          n153 = case shown="\"No Match\", Default" w358 {
            tunnel: ["End" "End" "End" "Meas Setups"] -> w357
            tunnel: [TRUE _ TRUE _] -> w356
            frame "No Match", Default {
            }
            frame "Meas Setups" {
              n154 = disable-structure shown="Disabled" {
                frame Disabled {
                  w364 = Setup_Filetype."Measurement Setups" ("Setup File Type")
                  w369 = string[] [] ("file names")
                  n155 = call "Last_Years_Setups.vi"("Setup File Type"=w364) -> ("Directory"=w363:path)
                  n156 = call "Setup_Filepath.vi"("Setup File Type"=w364, "Filename in"="Test") -> ("Directory"=w365:path)  [unwired: 1 out]
                  n157 = call "List_files_in_order_of_age.vi"("Files to Hide"=w369, "Folder"=w365) -> ("file names"=w366:string[])
                  n158 = call "List_files_in_order_of_age.vi"("Files to Hide"=w369, "Folder"=w363) -> ("file names"=w367:string[])
                  n159 = Build Array (concatenate)(w366, w367) -> ()  [unwired: 1 out]
                }
                frame Enabled {
                }
              }
              n160 = global write "Meas_global.vi" "Remote control"(FALSE ("Remote control")) -> ()
            }
            frame "End" {
            }
            frame "Load Subpanel" {
              n161 = property on="MRCMDFBGlobals" class="SubPnl"() -> (error out=w372:errorcluster, "InsertedVI"=w374:refnum<vi>)  [unwired: 2 in, 1 out]
              n162 = Not A Number/Path/Refnum?(number/path/refnum=w374) -> (NaN/Path/Refnum?=w373:bool)
              n163 = case shown="True" w373 {
                tunnel: w372 -> [_ w376]
                frame False {
                }
                frame True {
                  n164 = vi-ref "MRCMDFBGlobal.vi"() -> (w377:refnum<vi>)
                  n165 = invoke on="MRCMDFBGlobals" class="SubPnl" method="Insert VI"(error in=w376, "VI Ref"=w377) -> ()  [unwired: 2 in, 4 out]
                }
              }
            }
          }
        }
      }
      event Timeout {
        n166 = event-data() -> ()  [unwired: 1 in, 3 out]
      }
      event "Stop Button": Mouse Up {
        n167 = event-data() -> ()  [unwired: 1 in, 1 out]
        n168 = invoke on="MRCMDFBGlobals" class="SubPnl" method="Remove VI"() -> ()  [unwired: 3 in, 3 out]
      }
    }
  }
